vi "Memory Global.vi"() -> ()   [LabVIEW 2020]
panel:
  in  "Memory":T1(c390)
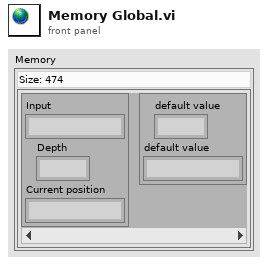
[diagram p1: front panel]
types:
  T1 = map{cluster{"Input":string, "Depth":u32, "Current position":string}, cluster{"default value":u64, "default value":string}}
diagram:
